vi "Handle Last Ack.vi"(8 "error in (no error)":errorcluster, 10 "Volatus:Module":refnum<class "Module.lvclass">, 11 "Volatus Core in":refnum<class "Volatus Core.lvclass">) -> (0 "error out":errorcluster, 1 "Close":bool, 3 "Volatus Core out":refnum<class "Volatus Core.lvclass">)   [LabVIEW 2020, in "Volatus.lvlib" / "Volatus Core.lvclass"]
uses:
  Volatus Core.lvclass
  C:/dev/lv20CE/relink/lv-volatus/Volatus/Module/Module.lvclass
  Module/Module.lvclass
  Reload State.ctl
  Volatus Core.lvclass/Volatus Core.ctl
  Module/Module.lvclass/Module.ctl
  MessageQ/MessageQ.lvclass
  MessageQ/MessageQ.lvclass/MessageQ.ctl
  MessageQ/Send.vi
  C:/dev/lv20CE/relink/lv-volatus/Volatus/Volatus Core/Volatus Core.lvclass
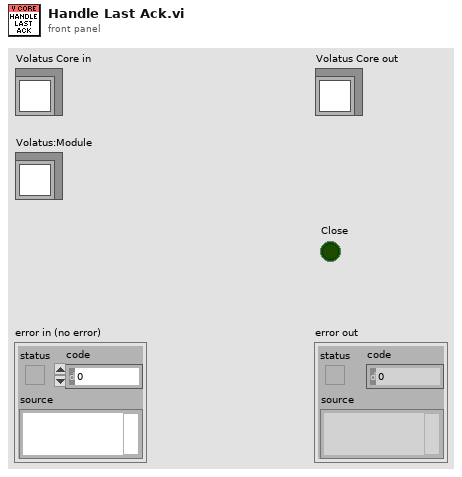
[diagram p1: front panel]
types:
  T1 = typedef "Volatus.lvlib/Volatus Core.lvclass/Reload State.ctl" = enum16{"None", "Stop Modules", "Close Vecto", "Reload", "Restart"}
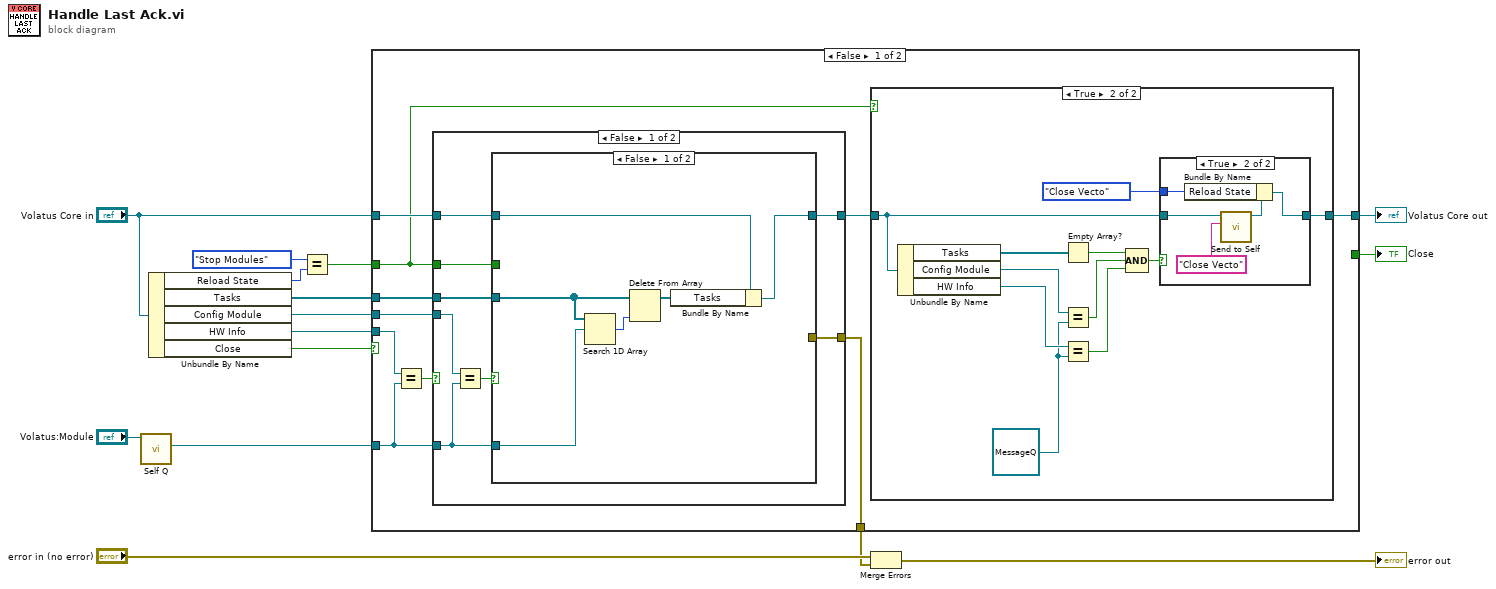
[diagram p0: block diagram]
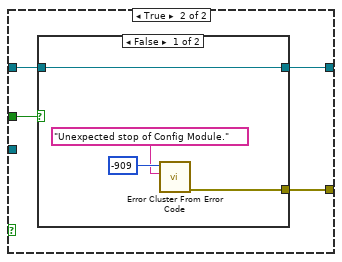
[diagram p2: hidden frame]
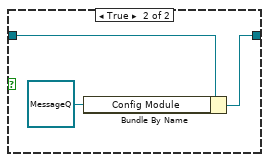
[diagram p3: hidden frame]
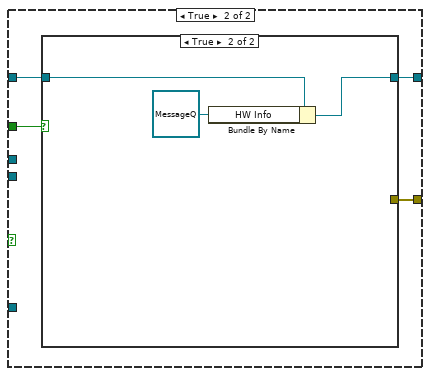
[diagram p4: hidden frame]
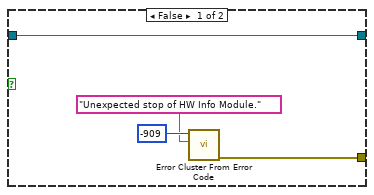
[diagram p5: hidden frame]
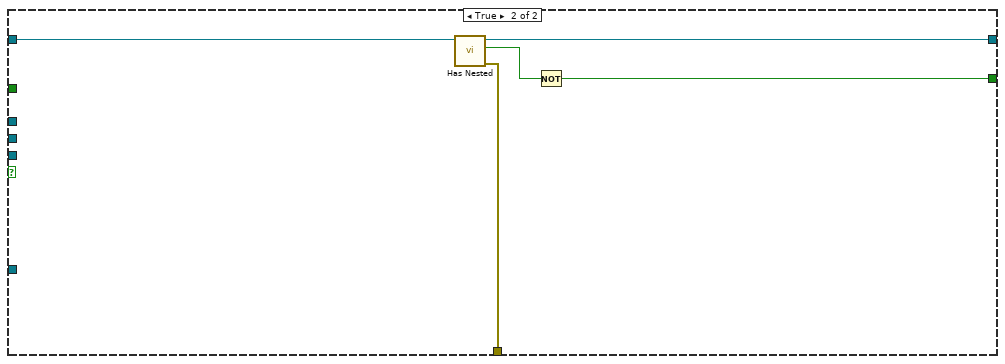
[diagram p8: hidden frame]
diagram:
  n1 = call "Self Q.vi"("Module in"="Volatus:Module") -> ("Self Q"=w3:refnum<class "MessageQ.lvclass">)  [unwired: 9 in, 1 out]
  n2 = Unbundle By Name("Volatus Core in") -> ("Reload State"=w12:T1, "Tasks"=w7:refnum<class "MessageQ.lvclass">[], "Config Module"=w13:refnum<class "MessageQ.lvclass">, "HW Info"=w4:refnum<class "MessageQ.lvclass">, "Close"=w2:bool)
  n3 = Equal?(x=Reload_State."Stop Modules", y=w12) -> (x = y?=w6:bool)
  n4 = case shown="False" w2 {
    tunnel: w13 -> [w25 _]
    tunnel: "Volatus Core in" -> [w24 w84]
    tunnel: [w23 w82] -> w8
    tunnel: w7 -> [w22 _]
    tunnel: w6 -> [w21 _]
    tunnel: [w19 w83] -> w5
    tunnel: w4 -> [w18 _]
    tunnel: w3 -> [w17 _]
    tunnel: [_ w80] -> w1
    frame False {
      n5 = Equal?(x=w18, y=w17) -> (x = y?=w16:bool)
      n6 = case shown="False" w16 {
        tunnel: w25 -> [w33 _]
        tunnel: w24 -> [w31 w52]
        tunnel: [w30 w54] -> w23
        tunnel: w17 -> [w29 _]
        tunnel: w22 -> [w28 _]
        tunnel: w21 -> [w27 w53]
        tunnel: [w26 w51] -> w20
        frame False {
          n7 = Equal?(x=w33, y=w29) -> (x = y?=w32:bool)
          n8 = case shown="False" w32 {
            tunnel: w27 -> [_ w41]
            tunnel: w31 -> [w39 w43]
            tunnel: [w38 w42] -> w26
            tunnel: [_ w40] -> w30
            tunnel: w29 -> [w36 _]
            tunnel: w28 -> [w37 _]
            frame False {
              n9 = Search 1D Array(1D array=w37, element=w36) -> (index of element=w35:i32)  [unwired: 1 in]
              n10 = Delete From Array(array=w37, index=w35) -> (array with subset deleted=w34:refnum<class "MessageQ.lvclass">[])  [unwired: 1 in, 1 out]
              n11 = Bundle By Name(cluster=w39, "Tasks"=w34) -> (w38:refnum<class "Volatus Core.lvclass">)
            }
            frame True {
              n12 = case shown="False" w41 {
                tunnel: w43 -> [w47 w50]
                tunnel: [w47 w49] -> w42
                tunnel: [w44 _] -> w40
                frame False {
                  n13 = call <vilib>:"Error Cluster From Error Code.vi"("error message (\"\")"="Unexpected stop of Config Module.", "error code (0)"=-909) -> ("error out"=w44:errorcluster)  [unwired: 7 in]
                }
                frame True {
                  n14 = Bundle By Name(cluster=w50, "Config Module"=refnum<class "MessageQ.lvclass"> refnum ("MsgQs.Config Module")) -> (w49:refnum<class "Volatus Core.lvclass">)
                }
              }
            }
          }
        }
        frame True {
          n15 = case shown="True" w53 {
            tunnel: [w56 _] -> w54
            tunnel: w52 -> [w55 w61]
            tunnel: [w55 w59] -> w51
            frame False {
              n16 = call <vilib>:"Error Cluster From Error Code.vi"("error message (\"\")"="Unexpected stop of HW Info Module.", "error code (0)"=-909) -> ("error out"=w56:errorcluster)  [unwired: 7 in]
            }
            frame True {
              n17 = Bundle By Name(cluster=w61, "HW Info"=refnum<class "MessageQ.lvclass"> refnum ("MsgQs.HW Info")) -> (w59:refnum<class "Volatus Core.lvclass">)
            }
          }
        }
      }
      n18 = case shown="True" w21 {
        tunnel: w20 -> [w62 w69]
        tunnel: [w62 w67] -> w19
        frame False {
        }
        frame True {
          w64 = refnum<class "MessageQ.lvclass"> refnum ("y")
          n19 = Unbundle By Name(w69) -> ("Tasks"=w72:refnum<class "MessageQ.lvclass">[], "Config Module"=w73:refnum<class "MessageQ.lvclass">, "HW Info"=w65:refnum<class "MessageQ.lvclass">)
          n20 = Empty Array?(array=w72) -> (empty?=w71:bool)
          n21 = Equal?(x=w73, y=w64) -> (x = y?=w70:bool)
          n22 = Equal?(x=w65, y=w64) -> (x = y?=w63:bool)
          n23 = Compound Arithmetic op=AND(w71, w70, w63) -> (w66:bool)
          n24 = case shown="True" w66 {
            tunnel: w69 -> [w74 w79]
            tunnel: Reload_State."Close Vecto" ("Reload State") -> [_ w77]
            tunnel: [w74 w76] -> w67
            frame False {
            }
            frame True {
              n25 = call "Send to Self.vi"("Message ID"="Close Vecto", "Module in"=w79) -> ("Module out"=w78:refnum<class "Volatus Core.lvclass">)  [unwired: 8 in, 1 out]
              n26 = Bundle By Name(cluster=w78, "Reload State"=w77) -> (w76:refnum<class "Volatus Core.lvclass">)
            }
          }
        }
      }
    }
    frame True {
      n27 = call "Has Nested.vi"("Module in"=w84) -> ("error out"=w82:errorcluster, "Has Nested"=w81:bool, "Module out"=w83:refnum<class "Volatus Core.lvclass">)  [unwired: 8 in]
      n28 = Not(x=w81) -> (.not. x?=w80:bool)
    }
  }
  "Volatus Core out" <- w5
  "Close" <- w1
  n29 = Merge Errors("error in (no error)", w8) -> (→"error out":errorcluster)
